vi "UI Refresh Data.vi"(8 "error in (no error)":errorcluster, 11 "GObject View in":refnum<class "RTM List View.lvclass">) -> (0 "error out":errorcluster, 3 "GObject View out":refnum<class "RTM List View.lvclass">)   [LabVIEW 2013, in "SET Project Editor.lvlib" / "RTM List View.lvclass"]
uses:
  RTM List View.lvclass
  RTM List View.lvclass/RTM List View.ctl
  UI View/UI View.lvclass/UI View.ctl
  SET Project Data/Project Data Class/Project Data.lvclass/Project Data.ctl
  SET Project Data/Menu Class/Menu Data.lvclass/Menu Data.ctl
  SET Project Data/Project Data Class/Read Menu Table.vi
  SET Project Data/Menu Class/Read Menu Path (Relative).vi
  SET Project Data/Menu Class/Read Menu Item LUT.vi
  UI View/Read _LangData.vi
  SET Project Editor.lvlib
  SET Project Data/Project Data Class/Project Data.lvclass
  SET Project Data/Menu Class/Menu Data.lvclass
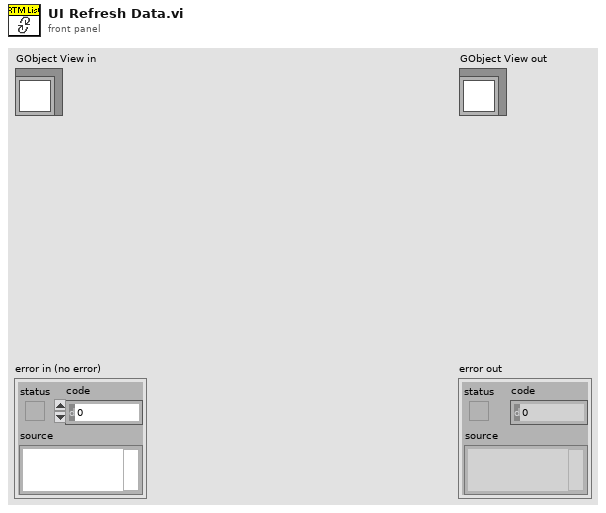
[diagram p1: front panel]
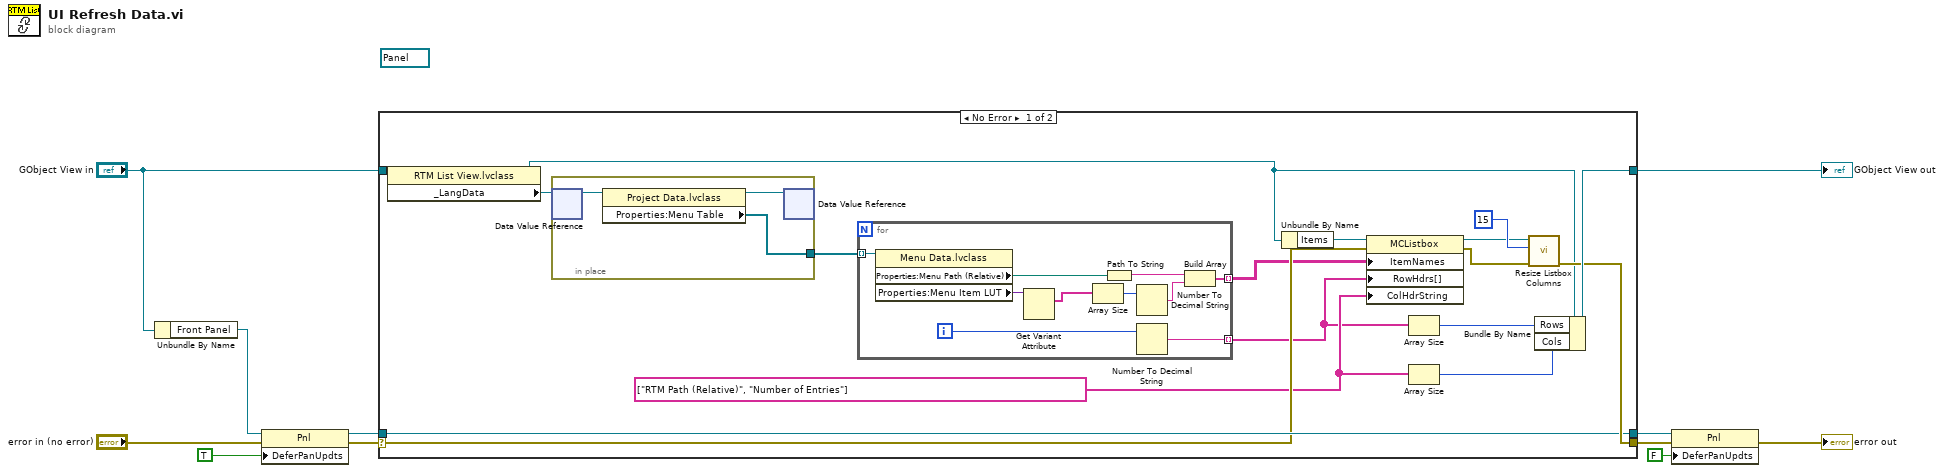
[diagram p0: block diagram]
diagram:
  (unwired) refnum<vi> refnum ("Front Panel")
  n1 = Unbundle By Name("GObject View in") -> ("Front Panel"=w9:refnum<vi>)
  n2 = property class="Pnl"(reference=w9, error in="error in (no error)", "DeferPanUpdts"=TRUE ("Defer Panel Updates")) -> (reference out=w5:refnum<vi>, error out=w6:errorcluster)
  n3 = case shown="No Error" w6 {
    selector: w6 -> [w19 w44]
    tunnel: [w24 w44] -> w3
    tunnel: [w28 w43] -> w11
    tunnel: "GObject View in" -> [w17 w43]
    tunnel: w5 -> [w21 w42]
    tunnel: [w21 w42] -> w4
    frame No Error {
      w18 = string[] ["RTM Path (Relative)", "Number of Entries"]
      n4 = property class="RTM List View.lvclass"(reference=w17) -> (reference out=w12:refnum<class "RTM List View.lvclass">, "_LangData"=w16:refnum<data-value>)  [unwired: 1 in, 1 out]
      n5 = in-place {
        in-place-border: [w29] -> w15
        n6 = in-place-dvr #1(w16) -> (w31:refnum<class "Project Data.lvclass">)  [unwired: 1 out]
        n7 = property class="Project Data.lvclass"(reference=w31) -> (reference out=w30:refnum<class "Project Data.lvclass">, "Properties:Menu Table"=w29:refnum<class "Menu Data.lvclass">[])  [unwired: 1 in, 1 out]
        n8 = in-place-dvr #1(w30) -> ()  [unwired: 2 out]
      }
      n9 = for {
        tunnel: w15 -> [w41] mode=indexing
        tunnel: [w36] -> w14 mode=indexing
        tunnel: [w34] -> w13 mode=indexing
        i -> [w35]
        n10 = property class="Menu Data.lvclass"(reference=w41) -> ("Properties:Menu Path (Relative)"=w40:path, "Properties:Menu Item LUT"=w33:variant)  [unwired: 1 in, 2 out]
        n11 = Get Variant Attribute(Variant=w33) -> (names=w32:string[])  [unwired: 3 in, 3 out]
        n12 = Array Size(array=w32) -> (size(s)=w39:i32)
        n13 = Path To String(path=w40) -> (string=w38:string)
        n14 = Number To Decimal String(number=w39) -> (decimal integer string=w37:string)  [unwired: 1 in]
        n15 = Number To Decimal String(number=w35) -> (decimal integer string=w34:string)  [unwired: 1 in]
        n16 = Build Array(w38, w37) -> (w36:string[])
      }
      n17 = Unbundle By Name(w12) -> ("Items"=w20:refnum<vi>)
      n18 = property class="MCListbox"(reference=w20, error in=w19, "ItemNames"=w14, "RowHdrs[]"=w13, "ColHdrString"=w18) -> (reference out=w26:refnum<vi>, error out=w25:errorcluster)
      n19 = Array Size(array=w13) -> (size(s)=w23:i32)
      n20 = Array Size(array=w18) -> (size(s)=w22:i32)
      n21 = call "Resize Listbox Columns.vi"("error in (no error)"=w25, "Padding (5px)"=i16 15, "Listbox Control ref in"=w26) -> ("error out"=w24:errorcluster)  [unwired: 7 in, 1 out]
      n22 = Bundle By Name(cluster=w12, "Rows"=w23, "Cols"=w22) -> (w28:refnum<class "RTM List View.lvclass">)
    }
    frame Error {
    }
  }
  "GObject View out" <- w11
  n23 = property class="Pnl"(reference=w4, error in=w3, "DeferPanUpdts"=FALSE ("Defer Panel Updates")) -> (error out=→"error out":errorcluster)  [unwired: 1 out]
